vi "Build_Write Multiple Coils.vi"(8 "error in (no error)":errorcluster, 9 "values":bool[](array[boolean]), 10 "starting address":u16) -> (0 "error out":errorcluster, 3 "MB_PDU":T1={"Function Code"=1, "Data"=[], "RTU_DataBytes"=0})   [LabVIEW 2021, in "MB Master.lvlib"]
doc: "Builds PDU for Write Multiple Coils (function code 15)."
uses:
  <vilib>/Plasmionique/MB Master/MB Master.lvlib
  <vilib>/Plasmionique/MB Master/MB_PDU/MB_PDU_Cluster.ctl
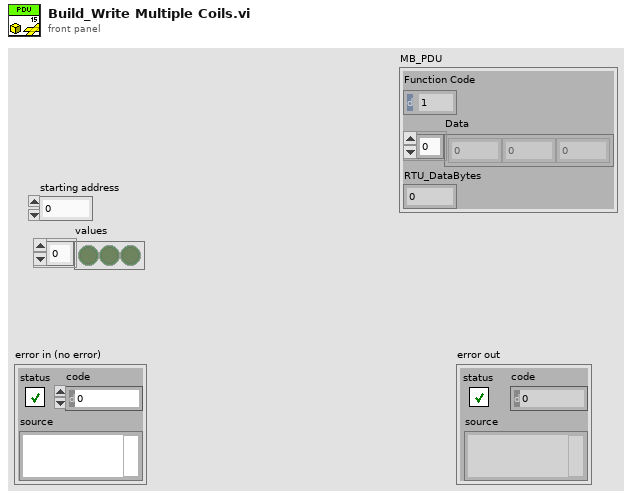
[diagram p1: front panel]
types:
  T1 = typedef "MB Master.lvlib/MB_PDU_Cluster.ctl" = cluster{"Function Code":u8, "Data":u8[], "RTU_DataBytes":i32}
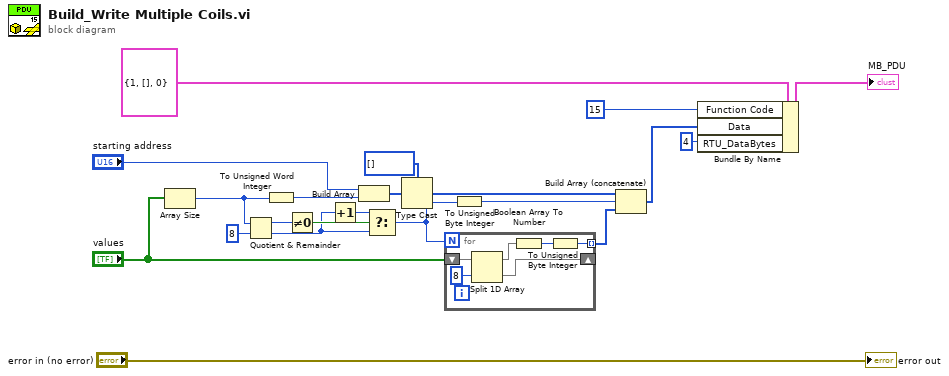
[diagram p0: block diagram]
diagram:
  n1 = Array Size(array="values") -> (size(s)=w5:i32)
  n2 = Quotient & Remainder(x=w5, y=8) -> (x-y*floor(x/y)=w11:i32, floor(x/y)=w8:i32)
  n3 = To Unsigned Word Integer(number=w5) -> (unsigned 16bit integer=w4:u16)
  n4 = Not Equal To 0?(x=w11) -> (x != 0?=w10:bool)
  n5 = Increment(x=w8) -> (x+1=w9:i32)
  n6 = Build Array("starting address", w4) -> (w21:u16[])
  n7 = Select(t=w9, s=w10, f=w8) -> (s? t:f=w3:i32)
  n8 = Type Cast(type=u8[] [], x=w21) -> (*(type *) &x=w14:u8[])
  n9 = for {
    N: w3 -> [_]
    shift-right: [w22] -> _
    shift-left: "values" -> [w27]
    tunnel: [w23] -> w7 mode=indexing
    n10 = Split 1D Array(array=w27, index=8) -> (first subarray=w24:bool[], second subarray=w22:bool[])
    n11 = Boolean Array To Number(Boolean array=w24) -> (number=w25:u32)
    n12 = To Unsigned Byte Integer(number=w25) -> (unsigned 8bit integer=w23:u8)
  }
  n13 = To Unsigned Byte Integer(number=w3) -> (unsigned 8bit integer=w2:u8)
  n14 = Build Array (concatenate)(w14, w2, w7) -> (w13:u8[])
  n15 = Bundle By Name(cluster=T1 {"Function Code"=1, "Data"=[], "RTU_DataBytes"=0} ("Modbus Serial New.lvlib:MB_PDU.lvclass"), "Function Code"=u8 15, "Data"=w13, "RTU_DataBytes"=4 ("NumBytes")) -> (→"MB_PDU":T1)
  "error out" <- "error in (no error)"
